vi "CoSim.vi"() -> ()   [LabVIEW 2015]
uses:
  AFE/Actions.ctl
  AFE/Gains.ctl
  AFE/Range.ctl
  AFE/Setpoint.ctl
  AFE/ManualControl.ctl
  AFE/Signals.ctl
  AFE/Parameters.ctl
  <vilib>/Simulation/Scripting/Companion Diagram/SimConfigNode/SimParams.ctl
  <vilib>/Simulation/Scripting/Companion Diagram/SimConfigNode/_simSolvers.ctl
  <vilib>/Simulation/Implementation/Shared/SIMSCR Execution Mode.ctl
  <vilib>/Simulation/Param Hierarchy/Typedefs/SIMPH Param Control Actions.ctl
  AFE/Inputs.ctl
  <vilib>/Simulation/Implementation/Shared/NILVSim_ParamChanged.vi
  <vilib>/Simulation/Implementation/Shared/NILVSIM_BeginStep.vi
  <vilib>/Simulation/Implementation/Shared/NILVSim_Manager.vi
  <vilib>/Utility/error.llb/Clear Errors.vi
  <vilib>/Simulation/Implementation/Shared/NILVSim_FinalizeModel.vi
  <vilib>/Simulation/Implementation/Shared/SIM Unbundle Sim Info.vi
  <vilib>/Simulation/Implementation/Shared/NILVSim_Initialize.vi
  <vilib>/NI/PowerElectronicsControl/Transforms/_IPBuilder/DeltaToWye_src.vi
  IPBuilder/AFE_SGL_src.vi
  LabVIEW 2015/IP Cores/IP Cores - LabVIEW FPGA/Control & Signal Gen/[FPGA] FXPT TriangleGen with Mod Index (use inside SCTL).vi
  LabVIEW 2015/IP Cores/IP Cores - LabVIEW FPGA/Control & Signal Gen/[FPGA] RIO Edge Delay (Use inside SCTL).vi
  <vilib>/Simulation/Utility/Implementation/NILVSim Get Time and IsAcceptedStep.vi
  <vilib>/Simulation/Implementation/Shared/SIMSH Read Queue.vi
  <vilib>/Simulation/Implementation/Shared/NILVSim_GetModelError.vi
  <vilib>/Simulation/Implementation/Shared/SIM Bundle Sim Info.vi
  <vilib>/Simulation/Scripting/Companion Diagram/SimConfigNode/SimDog.xnode
  <vilib>/Simulation/Implementation/XNodeFramework/SimXNode/SimX.xnode
  <vilib>/Simulation/EMI/Plugins/Multisim Design/MultisimEMICtrl.dll
  AFE/ActiveFrontEnd.lvlib
  <vilib>/Simulation/Implementation/Shared/NI_SIM_Implementation.lvlib
panel:
  in  "Mod Index (0..2)":fxp<+/-,32,2>
  in  "Carrier Freq":fxp<+/-,32,2>=0.00019999966025352478
  in  "Deadtime (=dT_s*40e6)":u32=40
  in  "Parameters":T1={"GridExpectedFreq"=60.0, "dT"=1e-05, "DirectIdCntrl"=FALSE, "AntiIslanding"=FALSE}
  out "VaCompare":dbl[][](graph)
  in  "Signals":T2
  in  "ManualControl":T3={"VDcmdEnable"=FALSE, "VDcmd"=1000.0, "VQcmdEnable"=FALSE, "VQcmd"=0.0, "IDcmdEnable"=FALSE, "IDcmd"=0.0, "IQcmdEnable"=FALSE, "IQcmd"=0.0}
  out "Calculated":sgl[][](graph)=[[391.9328, -0.010726929, -0.18300581, -7.3896046, 59.998215, 0.118336484]]
  in  "Setpoints":T4={"VDCLink"=2000.0, "DirectedIdSetpt"=0.0}
  in  "Range":T5={"PLL_PIRad_high"=140.0, "PLL_PiRad_low"=80.0, "IQcmd_high"=20.0, "IQcmd_low"=-20.0, "IDcmd_high"=40.0, "IDcmd_low"=-40.0, "VDcmd_high"=1200.0, "VDcmd_low"=0.0, "VQmcd_high"=500.0, "VQcmd_low"=-500.0}
  in  "Gains":T6={"PLL_proportional"=0.25, "PLL_integral"=0.0001, "antiIslanding_proportional"=0.0, "antiIslanding_integral"=0.0, "VDCLinkToID_proportional"=1.0, "VDCLinkToID_integral"=0.0001, "IDtoVD_proportional"=-5.0, "IDtoVD_integral"=-0.1, "IQtoVQ_proportional"=-5.0, "IQtoVQ_integral"=-0.01}
  out "Actions":T7={"PLL_proportional"=-0.0026817322, "PLL_integral"=119.99911, "antiIslanding_proportional"=-0.0, "antiIslanding_integral"=0.0, "VDCLink_proportional"=-696.84753, "VDCLink_integral"=-14.082889, "ID_proportional"=-199.08496, "ID_integral"=36.577522, "IQ_proportional"=36.94802, "IQ_integral"=463.09448}
  out "Currents":dbl[][](graph)=[[-0.6515756556764245, 2.540580686715224, -7.281866080538657, 4.741887768056174]]
  out "Voltages":dbl[][](graph)=[[1303.1499075060651, 364.6315309846368, -57.81778492642411, -306.8137219645202, -181.640625, 494.2336730957031, -312.5930480957031, 365.4536923916962, -59.331653509466776, -306.1218943280019]]
  in  "enable":bool
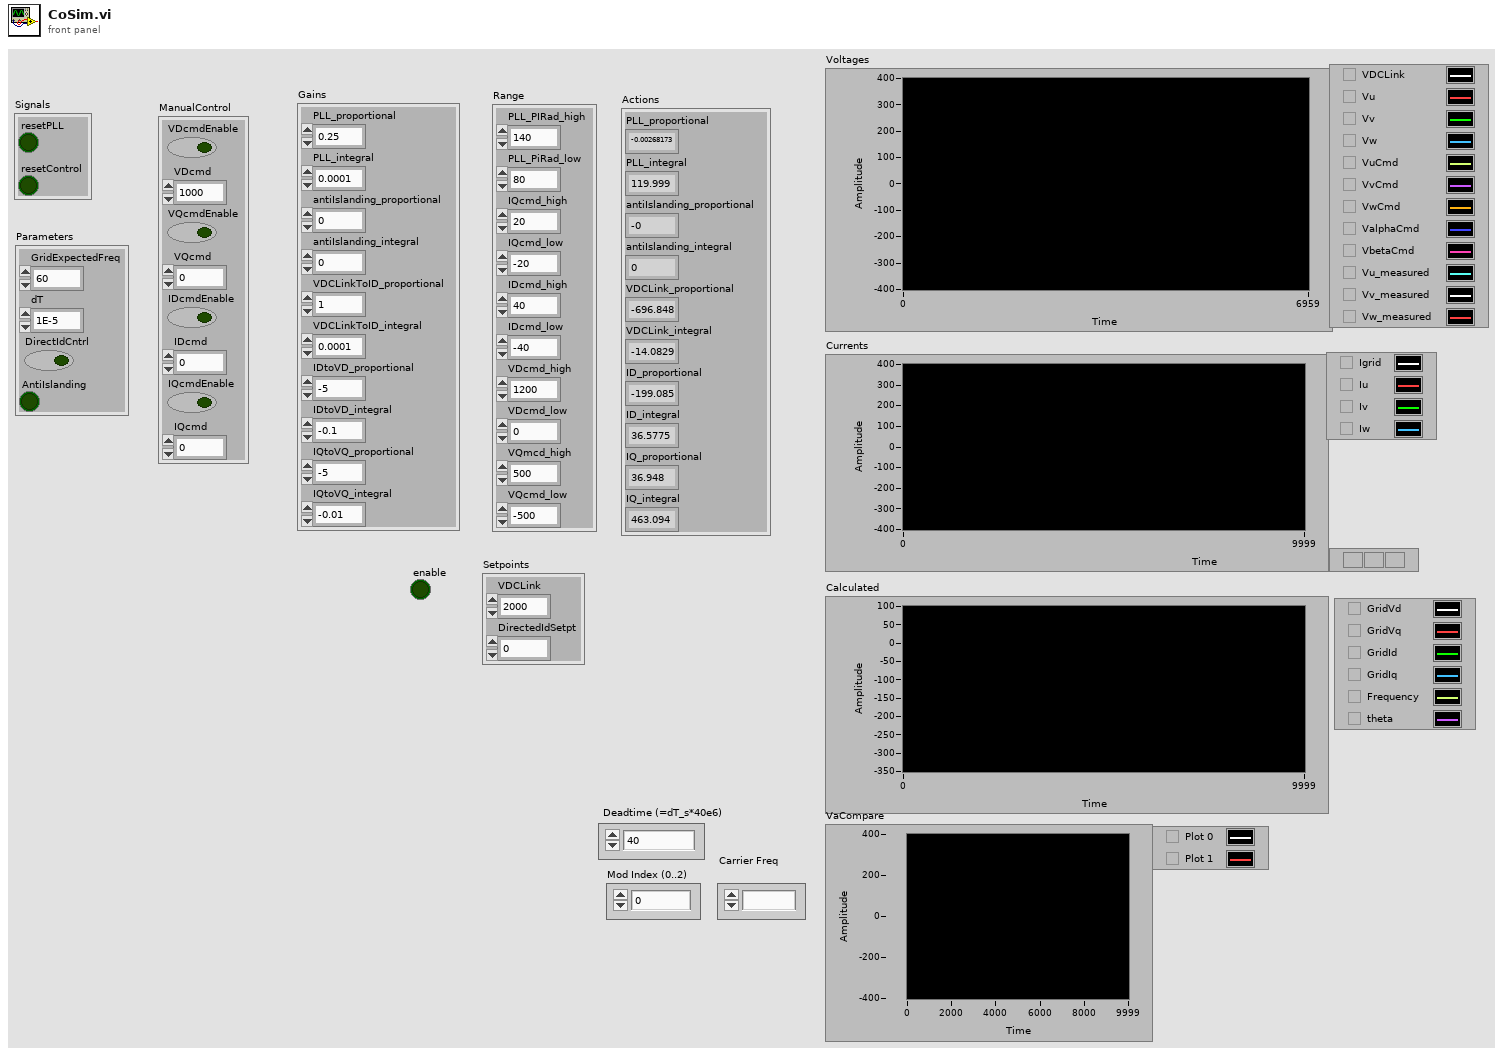
[diagram p1: front panel]
types:
  T1 = typedef "ActiveFrontEnd.lvlib/Parameters.ctl" = cluster{"GridExpectedFreq":sgl, "dT":sgl, "DirectIdCntrl":bool, "AntiIslanding":bool}
  T2 = typedef "ActiveFrontEnd.lvlib/Signals.ctl" = cluster{"resetPLL":bool, "resetControl":bool}
  T3 = typedef "ActiveFrontEnd.lvlib/ManualControl.ctl" = cluster{"VDcmdEnable":bool, "VDcmd":sgl, "VQcmdEnable":bool, "VQcmd":sgl, "IDcmdEnable":bool, "IDcmd":sgl, "IQcmdEnable":bool, "IQcmd":sgl}
  T4 = typedef "ActiveFrontEnd.lvlib/Setpoint.ctl" = cluster{"VDCLink":sgl, "DirectedIdSetpt":sgl}
  T5 = typedef "ActiveFrontEnd.lvlib/Range.ctl" = cluster{"PLL_PIRad_high":sgl, "PLL_PiRad_low":sgl, "IQcmd_high":sgl, "IQcmd_low":sgl, "IDcmd_high":sgl, "IDcmd_low":sgl, "VDcmd_high":sgl, "VDcmd_low":sgl, "VQmcd_high":sgl, "VQcmd_low":sgl}
  T6 = typedef "ActiveFrontEnd.lvlib/Gains.ctl" = cluster{"PLL_proportional":sgl, "PLL_integral":sgl, "antiIslanding_proportional":sgl, "antiIslanding_integral":sgl, "VDCLinkToID_proportional":sgl, "VDCLinkToID_integral":sgl, "IDtoVD_proportional":sgl, "IDtoVD_integral":sgl, "IQtoVQ_proportional":sgl, "IQtoVQ_integral":sgl}
  T7 = typedef "ActiveFrontEnd.lvlib/Actions.ctl" = cluster{"PLL_proportional":sgl, "PLL_integral":sgl, "antiIslanding_proportional":sgl, "antiIslanding_integral":sgl, "VDCLink_proportional":sgl, "VDCLink_integral":sgl, "ID_proportional":sgl, "ID_integral":sgl, "IQ_proportional":sgl, "IQ_integral":sgl}
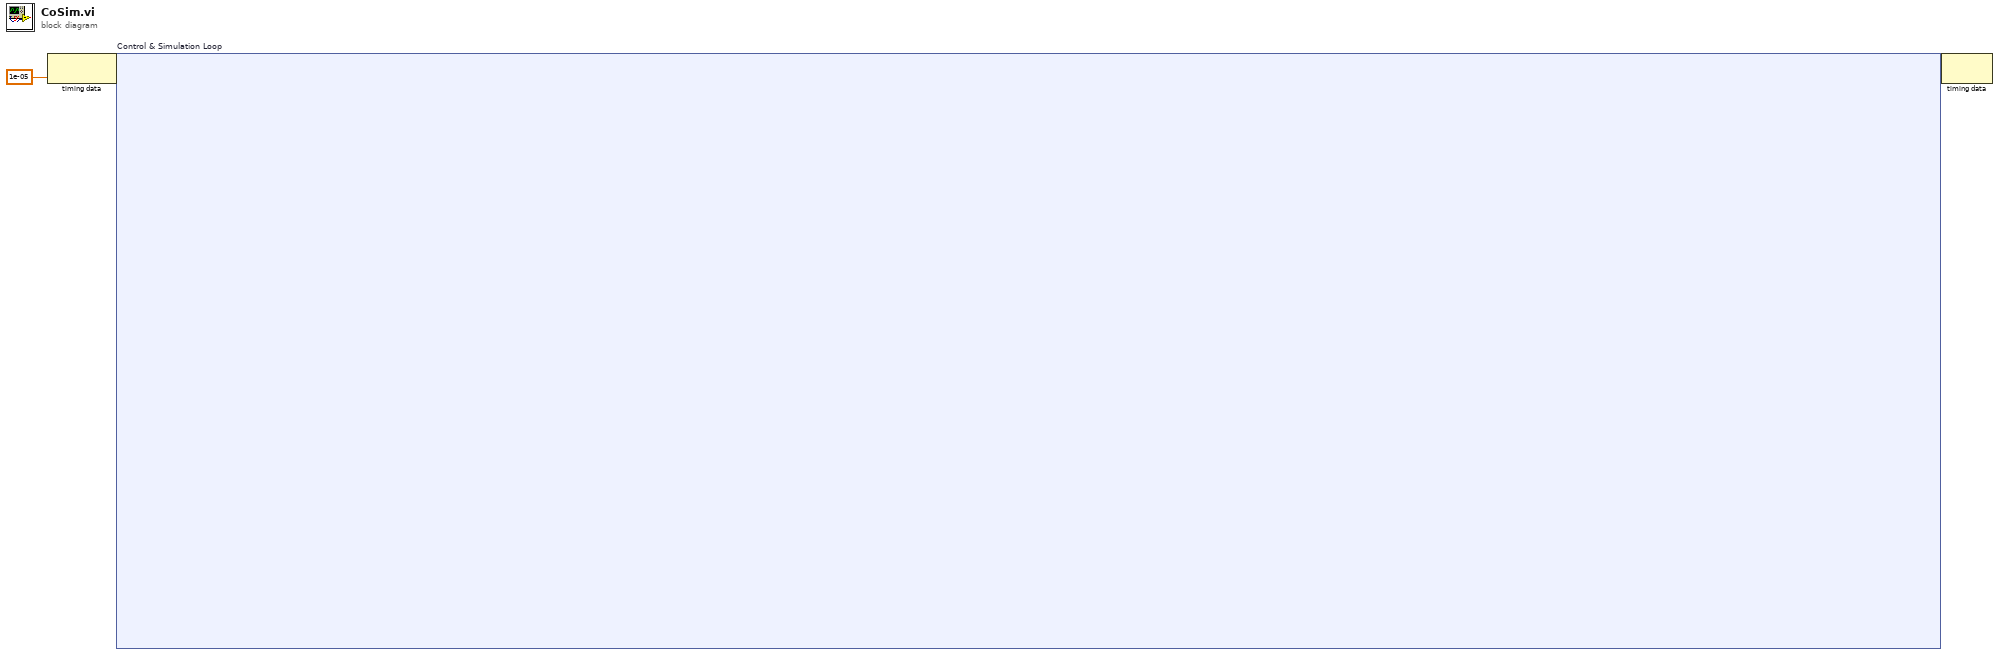
[diagram p0: block diagram]
diagram:
  n1 = node-c288(1e-05 ("Step Size (s)")) -> (w3:variant)
  n2 = node-c254 "Control & Simulation Loop"(w3) -> (w2:variant)
  n3 = node-c288(w2) -> ()  [unwired: 1 out]
